vi "Data Sorting 4 Sensor.vi"(0 "Data_Input":string) -> (1 "Data_Array Out":i32[](array[numeric]), 2 "SeqNum":u16, 3 "Battery_Voltage":dbl(knob) scale=0.0..3.0 scale format="%#3_3f", 4 "Sensor 1":i32[](array[numeric]), 5 "Sensor 2":i32[](array[numeric]), 6 "Sensor 3":i32[](array[numeric]), 7 "Sensor 4":i32[](array[numeric]))   [LabVIEW 2013]
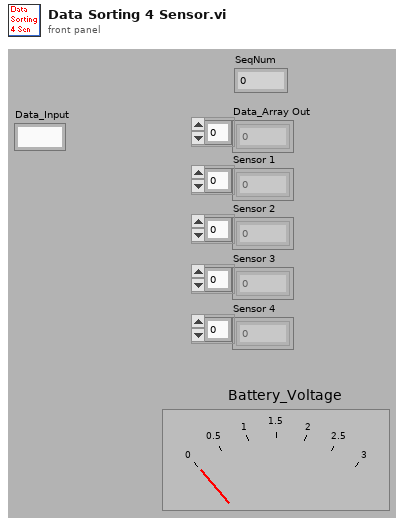
[diagram p1: front panel]
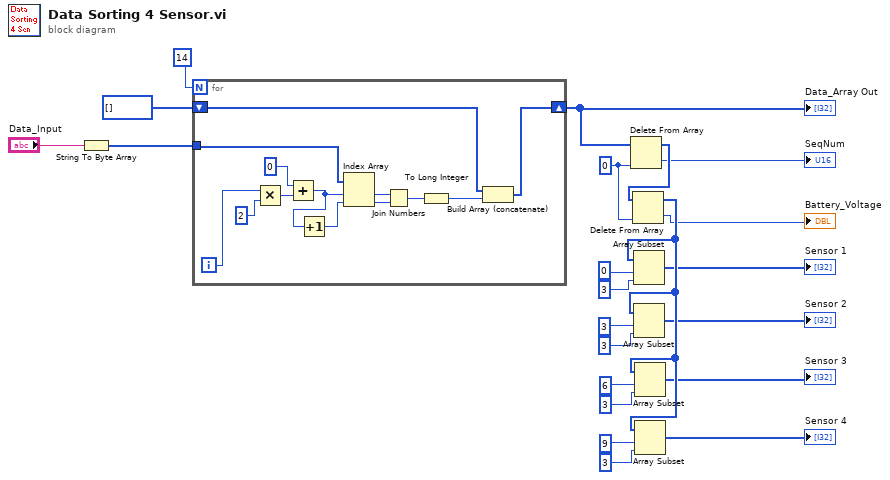
[diagram p0: block diagram]
diagram:
  w17 = 0
  n1 = String To Byte Array(string="Data_Input") -> (unsigned byte array=w21:u8[])
  n2 = for {
    N: 14 -> [_]
    tunnel: w21 -> [w34]
    shift-right: [w23] -> w14
    shift-left: i32[] [] -> [w24]
    i -> [w29]
    n3 = Multiply(x=w29, y=2) -> (x*y=w28:i32)
    n4 = Add(x=0, y=w28) -> (x+y=w26:i32)
    n5 = Increment(x=w26) -> (x+1=w33:i32)
    n6 = Index Array(array=w34, index #1=w26, index #2=w33) -> (element #1=w32:u8, element #2=w31:u8)
    n7 = Join Numbers(hi=w32, lo=w31) -> ((hi.lo)=w30:u16)
    n8 = To Long Integer(number=w30) -> (32bit integer=w27:i32)
    n9 = Build Array (concatenate)(w24, w27) -> (w23:i32[])
  }
  "Data_Array Out" <- w14
  n10 = Delete From Array(array=w14, index=w17) -> (deleted portion=→"SeqNum":i32, array with subset deleted=w18:i32[])  [unwired: 1 in]
  n11 = Delete From Array(array=w18, index=w17) -> (deleted portion=→"Battery_Voltage":i32, array with subset deleted=w7:i32[])  [unwired: 1 in]
  n12 = Array Subset(array=w7, index=0, length=3) -> (→"Sensor 1":i32[])
  n13 = Array Subset(array=w7, index=3, length=3) -> (→"Sensor 2":i32[])
  n14 = Array Subset(array=w7, index=6, length=3) -> (→"Sensor 3":i32[])
  n15 = Array Subset(array=w7, index=9, length=3) -> (→"Sensor 4":i32[])
